vi "Build Arduino Firmware.vi"() -> ()   [LabVIEW 2014]
panel:
  out "standard output":string
  out "standard error":string
  out "error out":errorcluster
  out "String":string
  in  "Arduino IDE Location":path
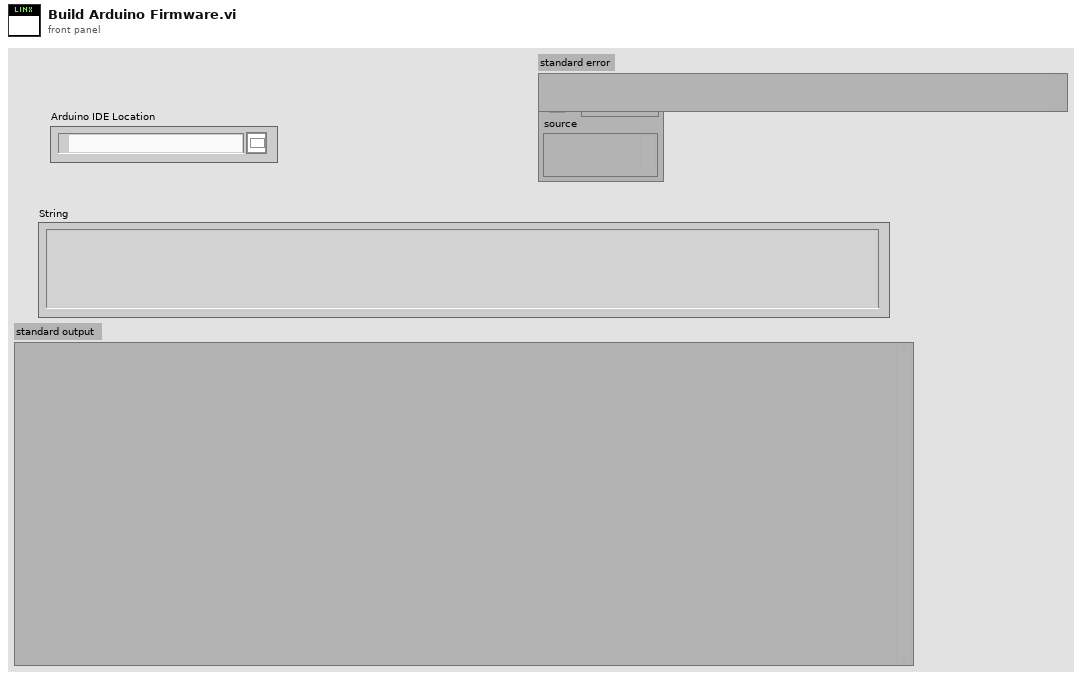
[diagram p1: front panel]
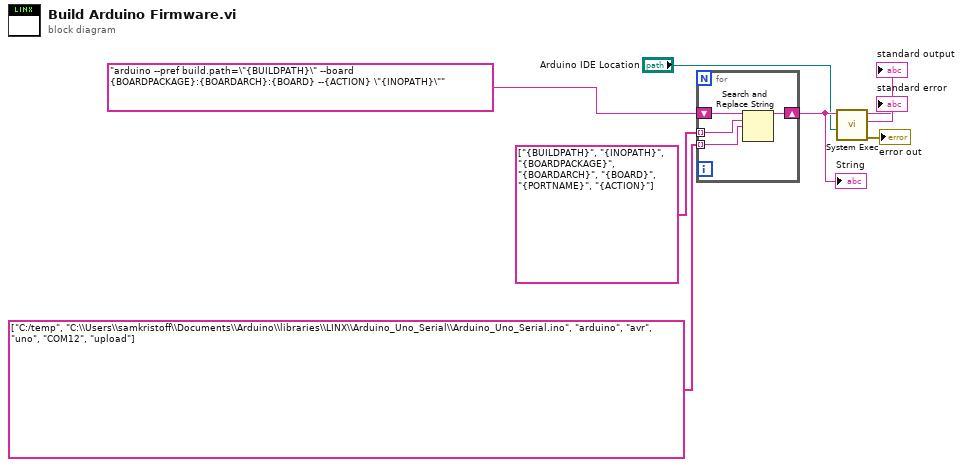
[diagram p0: block diagram]
diagram:
  n1 = for {
    shift-right: [w9] -> w5
    shift-left: "arduino --pref build.path=\"{BUILDPATH}\" --board {BOARDPACKAGE}:{BOARDARCH}:{BOARD} --{ACTION} \"{INOPATH}\"" -> [w12]
    tunnel: string[] ["{BUILDPATH}", "{INOPATH}", "{BOARDPACKAGE}", "{BOARDARCH}", "{BOARD}", "{PORTNAME}", "{ACTION}"] -> [w11] mode=indexing
    tunnel: string[] ["C:/temp", "C:\\Users\\samkristoff\\Documents\\Arduino\\libraries\\LINX\\Arduino_Uno_Serial\\Arduino_Uno_Serial.ino", "arduino", "avr", "uno", "COM12", "upload"] -> [w10] mode=indexing
    n2 = Search and Replace String(input string=w12, search string=w11, replace string=w10) -> (result string=w9:string)  [unwired: 5 in, 3 out]
  }
  "String" <- w5
  n3 = call <vilib>:"System Exec.vi"("working directory"="Arduino IDE Location", "command line"=w5) -> ("error out"=→"error out":errorcluster, "standard error"=→"standard error":string, "standard output"=→"standard output":string)  [unwired: 6 in, 1 out]
